vi "Boolean to Boolean String.vi"(0 "Boolean":bool, 1 "Force Lowercase? (t)":bool=TRUE) -> (2 "Boolean string":string)   [LabVIEW 2011]
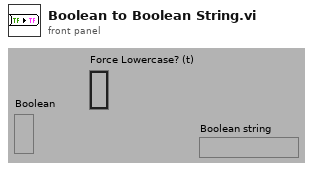
[diagram p1: front panel]
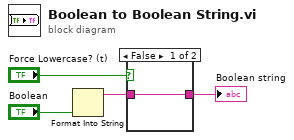
[diagram p0: block diagram]
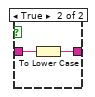
[diagram p2: hidden frame]
diagram:
  n1 = Format Into String("Boolean") -> (resulting string=w4:string)  [unwired: 3 in, 1 out]
  n2 = case shown="False" "Force Lowercase? (t)" {
    tunnel: w4 -> [w5 w7]
    tunnel: [w5 w6] -> w2
    frame False {
    }
    frame True {
      n3 = To Lower Case(string=w7) -> (all lower case string=w6:string)
    }
  }
  "Boolean string" <- w2
